vi "Scan Engine RT Driver.vi"(7 "Operation":T1, 11 "Device Reference in":T2 format="%.0x") -> (0 "Error Code":i32)   [LabVIEW 2016, in "Scan Engine Custom Device.lvlib"]
uses:
  Scan Engine Custom Device.lvlib
  <vilib>/NI Veristand/Custom Device API/Custom Device Item Ref.ctl
  <vilib>/NI Veristand/Custom Device API/Hardware Interface Driver VI Operation.ctl
  Type Defs/RT Data.ctl
  Type Defs/Device Channels.ctl
  Type Defs/Output Data.ctl
  <vilib>/NI Veristand/Custom Device API/Block Data Reference.ctl
  <vilib>/NI Veristand/Custom Device API/Data Reference.ctl
  Type Defs/Input Data.ctl
  Type Defs/Local Chassis Data.ctl
  Type Defs/RSI Module Data.ctl
  Type Defs/Open Module IOVs.ctl
  Modules.lvlibp/RSI Module/RSI Module.lvclass
  Modules.lvlibp/RSI Module/Module Models.ctl
  Modules.lvlibp/RSI Module/Channel Type.ctl
  Type Defs/Module Config Data.ctl
  Type Defs/Mixed IO.ctl
  Type Defs/FPGA Data.ctl
  Type Defs/UDV Data.ctl
  Type Defs/UDV Data Type.ctl
  Type Defs/FXP Config.ctl
  Type Defs/Mod Size Indexes.ctl
  Type Defs/EtherCAT Master Data.ctl
  Type Defs/EtherCAT Slave Data.ctl
  Type Defs/Generic ECAT Slave RT-Data-Array.ctl
  Type Defs/Generic ECAT Slave Data Cluster.ctl
  Type Defs/Generic ECAT Slave IOV Cluster.ctl
  Type Defs/Async Data.ctl
  Type Defs/Async Status.ctl
  Type Defs/Async State.ctl
  Type Defs/Async Command.ctl
  Type Defs/ECAT Reconfig Data.ctl
  Type Defs/ECAT Reconfig Status.ctl
  Type Defs/ECAT Reconfig State.ctl
  Async/Get Async Status.vi
  Utility/Set Error.vi
  Read-Write/RW All Data.vi
  Read-Write/RW All Local.vi
  Read-Write/RW All ECAT.vi
  Read-Write/Check Command Channels.vi
  Read-Write/Read Async FIFOs.vi
  Read-Write/Update Status Channels.vi
  Module Reconfig/Check ECAT Reconfig.vi
  Read-Write/Write Async FIFOs.vi
  Read-Write/RW Local Chassis.vi
  Read-Write/RW Slave.vi
  Read-Write/RW Generic Slaves.vi
  <vilib>/NI Veristand/Custom Device API/NI VeriStand - Get Channel Values by Block Data Reference.vi
  <vilib>/NI Veristand/Custom Device API/NI VeriStand - Set Channel Values by Block Data Reference.vi
  Read-Write/RW UDVs.vi
  Read-Write/RW Mods.vi
  Read-Write/Read ECAT VARs.vi
  Read-Write/Write ECAT VARs.vi
  Read-Write/Read UDVs.vi
  Read-Write/Write UDVs.vi
  Read-Write/Read All Input Module Sizes.vi
  Read-Write/Read All Mixed Module Sizes.vi
  Read-Write/Write Module.vi
  Read-Write/Check Module Config.vi
  Read-Write/Scanned Read - UDV.vi
  Read-Write/Scanned Write - UDV.vi
  Read-Write/Read Input Modules at Indexes.vi
  Read-Write/Read Mixed Modules at Indexes.vi
  Read-Write/Scanned Write - Module.vi
  Read-Write/Read Input Module.vi
  Read-Write/Read Mixed Module.vi
  Read-Write/Scanned Read - Input Module.vi
  Read-Write/Scanned Read - Mixed Module.vi
  <vilib>/NI Veristand/Custom Device API/Global Data Refs.vi
  Module Reconfig/Set ECAT Reconfig Status.vi
  Read-Write/Launch Local Reconfig.vi
  Async/Set Async Status.vi
  Read-Write/Launch ECAT Reconfig.vi
  Globals/Error Strings.vi
  Module Reconfig/Get ECAT Reconfig Status.vi
  Read-Write/Get Scan Mode.vi
  <vilib>/Utility/error.llb/Error Cluster From Error Code.vi
  <vilib>/NI Veristand/Custom Device API/Custom Device API.lvlib
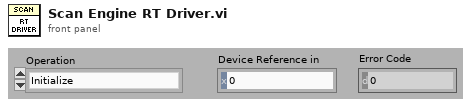
[diagram p1: front panel]
types:
  T1 = typedef "Custom Device API.lvlib/Hardware Interface Driver VI Operation.ctl" = enum16{"Initialize", "Start", "Read Data from HW", "Write Data to HW", "Close"}
  T2 = typedef "Custom Device API.lvlib/Custom Device Item Ref.ctl" = u64
  T3 = typedef "Scan Engine Custom Device.lvlib/RT Data.ctl" = cluster{"Device ref":T2, "Scan Period (uSec)":u32, "Device Channels":T4, "Local Chassis":T9[], "EtherCAT Masters":T21[], "Async":T26, "ECAT Reconfig":T27, "Device Error":errorcluster, "DeviceName":string, "PCLSync?":bool}
  T4 = typedef "Scan Engine Custom Device.lvlib/Device Channels.ctl" = cluster{"Status":T5, "Command":T8}
  T5 = typedef "Scan Engine Custom Device.lvlib/Output Data.ctl" = cluster{"BD Refs":T6[], "Length":i32, "FIFO Index":i32, "Data":dbl[]}
  T6 = typedef "Custom Device API.lvlib/Block Data Reference.ctl" = cluster{"Data Reference":T7, "Offset":u64, "Length":u64}
  T7 = typedef "Custom Device API.lvlib/Data Reference.ctl" = i32
  T8 = typedef "Scan Engine Custom Device.lvlib/Input Data.ctl" = cluster{"BD Refs":T6[], "Data":dbl[], "Length":i32, "FIFO Index":i32}
  T9 = typedef "Scan Engine Custom Device.lvlib/Local Chassis Data.ctl" = cluster{"VS ref":T2, "RSI Modules":T10[], "FPGA":T16[], "Input Mod Size Idxs":T20, "Output Modules":i32[], "MixedIO Mod Size Idxs":T20}
  T10 = typedef "Scan Engine Custom Device.lvlib/RSI Module Data.ctl" = cluster{"VS ref":T2, "IOV ref":refnum<k21>, "Open Mod refs":T11, "Module DVR":refnum<data-value>, "Slot":u32, "Model":T12, "Channel Type":T13, "EtherCAT?":bool, "CDInput Data":T8, "CDOutput Data":T5, "Module Config Data":T14, "Mixed IO":T15}
  T11 = typedef "Scan Engine Custom Device.lvlib/Open Module IOVs.ctl" = cluster{"Analog Read":refnum<k21>, "Digital Read":refnum<k21>, "Analog Write":refnum<k21>, "Digital Write":refnum<k21>}
  T12 = typedef "Modules.lvlibp/RSI Module.lvclass/Module Models.ctl" = enum16{"Empty", "NI 9201", "NI 9203", "NI 9205", "NI 9206", "NI 9207", "NI 9208", "NI 9211", "NI 9212", "NI 9213", "NI 9214", "NI 9215", "NI 9217", "NI 9219", "NI 9220", "NI 9221", "NI 9222", "NI 9223", "NI 9225", "NI 9227", "NI 9229", "NI 9233", "NI 9234", "NI 9235", "NI 9236", "NI 9237", "NI 9239", "NI 9242", "NI 9244", "NI 9263", "NI 9264", "NI 9265", "NI 9269", "NI 9375", "NI 9401", "NI 9402", "NI 9403", "NI 9411", "NI 9421", "NI 9422", "NI 9423", "NI 9425", "NI 9426", "NI 9435", "NI 9437", "NI 9472", "NI 9474", "NI 9475", "NI 9476", "NI 9477", "NI 9478", "NI 9481", "NI 9482", "NI 9485"}
  T13 = typedef "Modules.lvlibp/RSI Module.lvclass/Channel Type.ctl" = enum16{"Analog", "Digital"}
  T14 = typedef "Scan Engine Custom Device.lvlib/Module Config Data.ctl" = cluster{"Configurable?":bool, "Config Block Data Refs":T6[], "Config Data DVR":refnum<data-value>, "Previous Values":dbl[], "Local Reconfig VI Ref":refnum<vi>}
  T15 = typedef "Scan Engine Custom Device.lvlib/Mixed IO.ctl" = cluster{"Input Channel Indices":i32[], "Input Buffer":dbl[]}
  T16 = typedef "Scan Engine Custom Device.lvlib/FPGA Data.ctl" = cluster{"VS ref":T2, "IOV ref":refnum<k21>, "FPGA Target":enum16{"Local", "EtherCAT"}, "Product Code":u32, "Bitfile Signature":string, "Bitfile Path (RT)":path, "FPGA Session":u32, "Input Data":T8, "Output Data":T5, "UDVs":cluster{"From FPGA":T17[], "To FPGA":T17[]}}
  T17 = typedef "Scan Engine Custom Device.lvlib/UDV Data.ctl" = cluster{"VS ref":T2, "IOV Ref":refnum<k21>, "Name":string, "UDV Data Type":T18, "Supported Type?":bool, "FXP Config":T19, "FXP VI Ref":refnum<vi>}
  T18 = typedef "Scan Engine Custom Device.lvlib/UDV Data Type.ctl" = enum16{"Boolean", "Fixed Point", "Int8", "Int16", "Int32", "Int64", "U32 Bit Field", "UInt8", "UInt16", "UInt32", "UInt64", "Other"}
  T19 = typedef "Scan Engine Custom Device.lvlib/FXP Config.ctl" = cluster{"signed":bool, "size":u32, "integersize":i32}
  T20 = typedef "Scan Engine Custom Device.lvlib/Mod Size Indexes.ctl" = cluster{"4":i32[], "8":i32[], "16":i32[], "32":i32[], "other":i32[]}
  T21 = typedef "Scan Engine Custom Device.lvlib/EtherCAT Master Data.ctl" = cluster{"VS ref":T2, "IOV ref":refnum<k21>, "Master ID":u32, "Cyclic Data Bandwidth":u32, "EtherCAT Slaves":T22[], "Generic EtherCAT Slaves":T23}
  T22 = typedef "Scan Engine Custom Device.lvlib/EtherCAT Slave Data.ctl" = cluster{"VS ref":T2, "IOV ref":refnum<k21>, "Position Address":u16, "RSI Modules":T10[], "FPGA":T16[], "Input Mod Size Idxs":T20, "Output Modules":i32[], "MixedIO Mod Size Idxs":T20}
  T23 = typedef "Scan Engine Custom Device.lvlib/Generic ECAT Slave RT-Data-Array.ctl" = T24[]
  T24 = typedef "Scan Engine Custom Device.lvlib/Generic ECAT Slave Data Cluster.ctl" = cluster{"VS ref":T2, "IOV ref":refnum<k21>, "Position Address":u16, "I/O Imput Vars ":T25[], "I/O Output Vars":T25[], "I/O Input Data":T8, "I/O Output Data":T5}
  T25 = typedef "Scan Engine Custom Device.lvlib/Generic ECAT Slave IOV Cluster.ctl" = cluster{"VS ref":T2, "IOV Ref":refnum<k21>, "Name":string, "UDV Data Type":T18}
  T26 = typedef "Scan Engine Custom Device.lvlib/Async Data.ctl" = cluster{"Status":refnum<queue>, "Command":refnum<queue>, "Input FIFO":refnum<k33>, "Input FIFO buffer":dbl[], "Output FIFO":refnum<k33>, "Output FIFO buffer":dbl[], "Async VI Ref":refnum<vi>}
  T27 = typedef "Scan Engine Custom Device.lvlib/ECAT Reconfig Data.ctl" = cluster{"Reconfig Module Found":bool, "VI Ref":refnum<vi>, "Status":refnum<queue>}
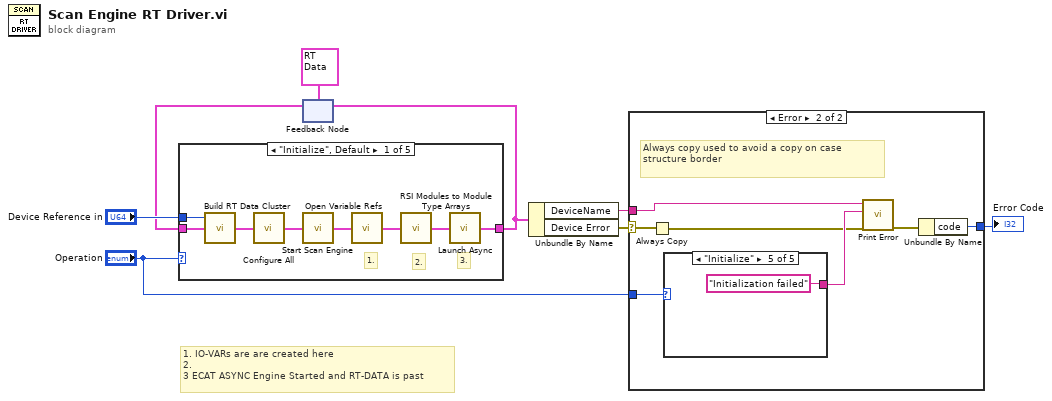
[diagram p0: block diagram]
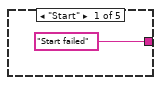
[diagram p3: hidden frame]
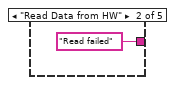
[diagram p4: hidden frame]
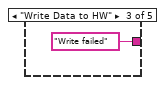
[diagram p5: hidden frame]
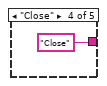
[diagram p6: hidden frame]
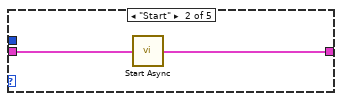
[diagram p7: hidden frame]
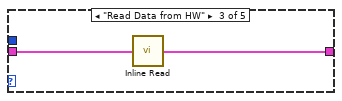
[diagram p8: hidden frame]
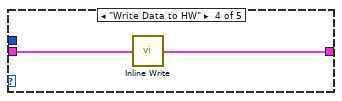
[diagram p9: hidden frame]
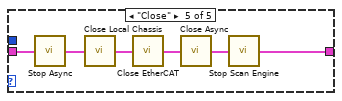
[diagram p10: hidden frame]
diagram:
  # "1. IO-VARs are are created here\n2.\n3 ECAT ASYNC Engine Started and RT-DATA is past"
  n1 = feedback #1(T3 {"Device ref"=0, "Scan Period (uSec)"=0, "Device Channels"={"Status"={"BD Refs"=[], "Length"=0, "FIFO Index"=0, "Data"=[]}, "Command"={"BD Refs"=[], "Data"=[], "Length"=0, "FIFO Index"=0}}, "Local Chassis"=[], "EtherCAT Masters"=[], "Async"={"Status"=refnum, "Command"=refnum, "Input FIFO"=refnum, "Input FIFO buffer"=[], "Output FIFO"=refnum, "Output FIFO buffer"=[], "Async VI Ref"=refnum}, "ECAT Reconfig"={"Reconfig Module Found"=FALSE, "VI Ref"=refnum, "Status"=refnum}, "Device Error"={"status"=FALSE, "code"=0, "source"=""}, "DeviceName"="", "PCLSync?"=FALSE} ("RT Data")) -> (w6:T3)
  n2 = case shown="\"Initialize\", Default" "Operation" {
    tunnel: "Device Reference in" -> [w16 _ _ _ _]
    tunnel: w6 -> [w14 w18 w20 w21 w28]
    tunnel: [w10 w17 w19 w22 w23] -> w4
    frame "Initialize", Default {
      # "3."
      # "2."
      # "1."
      n3 = call "Build RT Data Cluster.vi"("Device Reference in"=w16, "RT Data in"=w14) -> ("RT Data out"=w15:T3)  [unwired: 7 in]
      n4 = call "Configure All.vi"("RT Data in"=w15) -> ("RT Data out"=w13:T3)
      n5 = call "Start Scan Engine.vi"("RT Data in"=w13) -> ("RT Data out"=w12:T3)
      n6 = call "Open Variable Refs.vi"("RT Data in"=w12) -> ("RT Data out"=w11:T3)
      n7 = call "RSI Modules to Module Type Arrays.vi"("RT Data in"=w11) -> ("RT Data out"=w9:T3)
      n8 = call "Launch Async.vi"("RT Data in"=w9) -> ("RT Data out"=w10:T3)
    }
    frame "Start" {
      n9 = call "Start Async.vi"("RT Data in"=w18) -> ("RT Data out"=w17:T3)
    }
    frame "Read Data from HW" {
      n10 = call "Inline Read.vi"("RT Data in"=w20) -> ("RT Data out"=w19:T3)
    }
    frame "Write Data to HW" {
      n11 = call "Inline Write.vi"("RT Data"=w21) -> ("RT Data out"=w22:T3)
    }
    frame "Close" {
      n12 = call "Stop Async.vi"("RT Data in"=w28) -> ("RT Data out"=w25:T3)
      n13 = call "Close Local Chassis.vi"("RT Data in"=w25) -> ("RT Data out"=w27:T3)
      n14 = call "Close EtherCAT.vi"("RT Data in"=w27) -> ("RT Data out"=w26:T3)
      n15 = call "Close Async.vi"("RT Data in"=w26) -> ("RT Data out"=w24:T3)
      n16 = call "Stop Scan Engine.vi"("RT Data in"=w24) -> ("RT Data out"=w23:T3)
    }
  }
  n17 = feedback-in #1(w4) -> ()
  n18 = Unbundle By Name(w4) -> ("DeviceName"=w2:string, "Device Error"=w3:errorcluster)
  n19 = case shown="Error" w3 {
    selector: w3 -> [_ w34]
    tunnel: [_ w29] -> w8
    tunnel: w2 -> [_ w33]
    tunnel: "Operation" -> [_ w32]
    frame No Error {
      # "Don't send warnings"
    }
    frame Error {
      # "Always copy used to avoid a copy on case structure border"
      n20 = Always Copy(1:w34) -> (0:w30:errorcluster)
      n21 = case shown="\"Initialize\"" w32 {
        tunnel: ["Start failed" ("Note (empty)") "Read failed" ("Note (empty)") "Write failed" ("Note (empty)") "Close" ("Note (empty)") "Initialization failed" ("Note (empty)")] -> w31
        frame "Start" {
        }
        frame "Read Data from HW" {
        }
        frame "Write Data to HW" {
        }
        frame "Close" {
        }
        frame "Initialize" {
        }
      }
      n22 = call "Print Error.vi"("error in (no error)"=w30, "Note (empty)"=w31, "Your code's public name"=w33) -> ("error out"=w35:errorcluster)  [unwired: 7 in]
      n23 = Unbundle By Name(w35) -> ("code"=w29:i32)
    }
  }
  "Error Code" <- w8
